vi "全局 1.vi"() -> ()   [LabVIEW 2014]
panel:
  in  "列":i32
  in  "雷":i32
  in  "行":i32
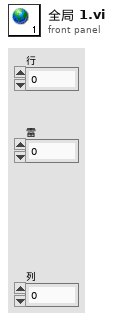
[diagram p1: front panel]
diagram:
